vi "Read Tau Data off U.vi"() -> ()   [LabVIEW 2012]
panel:
  out "size(s)":i32
  out "Waveform Graph":sgl[](graph)
  out "appended array":timestamp[](array[timestamp])
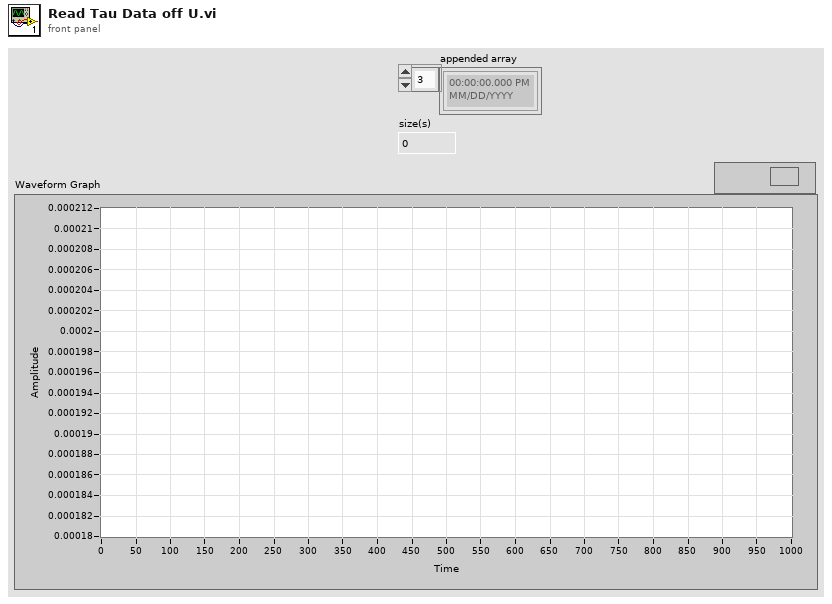
[diagram p1: front panel]
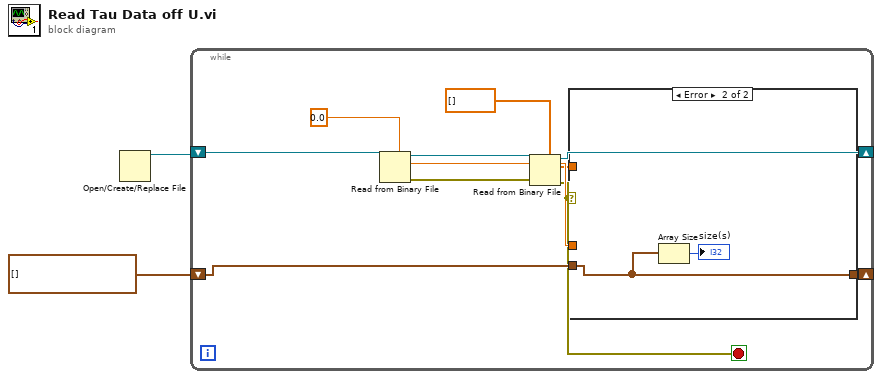
[diagram p0: block diagram]
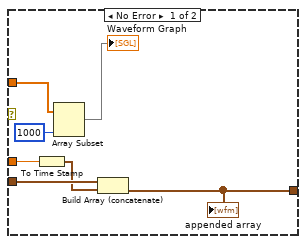
[diagram p2: hidden frame]
diagram:
  n1 = Open/Create/Replace File() -> (refnum out=w1:refnum<file>)  [unwired: 6 in, 2 out]
  n2 = while {
    shift-right: [w10] -> _
    shift-left: w1 -> [w13]
    shift-right: [w5] -> _
    shift-left: timestamp[] [] -> [w6]
    stop <- w3 stop-if-true
    n3 = Read from Binary File(5:0.0, 11:w13) -> (0:w9:errorcluster, 2:w7:dbl, 3:w11:refnum<file>)  [unwired: 4 in, 1 out]
    n4 = Read from Binary File(5:sgl[] [], 8:w9, 11:w11) -> (0:w3:errorcluster, 2:w4:sgl[], 3:w10:refnum<file>)  [unwired: 3 in, 1 out]
    n5 = case shown="Error" w3 {
      tunnel: w7 -> [w20 _]
      tunnel: w6 -> [w19 w22]
      tunnel: [w17 w22] -> w5
      tunnel: w4 -> [w16 _]
      frame No Error {
        n6 = To Time Stamp(1:w20) -> (0:w18:timestamp)
        n7 = Array Subset(array=w16, length=1000) -> (→"Waveform Graph":sgl[])  [unwired: 1 in]
        n8 = Build Array (concatenate)(w19, w18) -> (w17:timestamp[])
        "appended array" <- w17
      }
      frame Error {
        n9 = Array Size(array=w22) -> (size(s)=→"size(s)":i32)
      }
    }
  }
